vi "Activity_10.vi"() -> ()   [LabVIEW 2015]
panel:
  out "10<Num<30":dbl[](array[numeric])
  out "Array":dbl[](array[numeric])
  out "Num.\nAleatorio":dbl
  out "Iteracion":i32
  # "Selector de números aleatorios en un rango"
  # "Serrano Bermúdez Luis Esteban\nFecha de Entrega 23/02/2019"
  # "Descripción:"
  # "Genera 10 números aleatorios y elige entre un rango de\nvalores determinado (para este ejercicio los valores elegidos\nson 10<Num<30)"
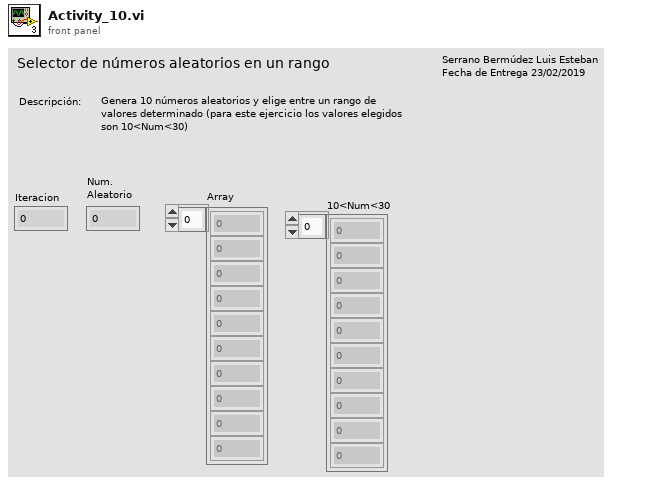
[diagram p1: front panel]
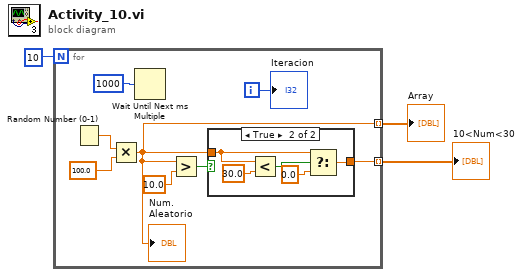
[diagram p0: block diagram]
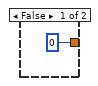
[diagram p2: hidden frame]
diagram:
  n1 = for {
    N: 10 -> [_]
    tunnel: [w5] -> w2 mode=indexing
    tunnel: [w4] -> w1 mode=indexing
    i -> [w11]
    n2 = Random Number (0-1)() -> (number: 0 to 1=w9:dbl)
    n3 = Multiply(x=w9, y=100.0) -> (x*y=w5:dbl)
    "Num.\nAleatorio" <- w5
    n4 = Wait Until Next ms Multiple(millisecond multiple=u32 1000) -> ()  [unwired: 1 out]
    n5 = Greater?(x=w5, y=10.0) -> (0:w6:bool)
    n6 = case shown="True" w6 {
      tunnel: w5 -> [_ w15]
      tunnel: [0 w14] -> w4
      frame False {
      }
      frame True {
        n7 = Less?(x=w15, y=30.0) -> (x < y?=w16:bool)
        n8 = Select(t=w15, s=w16, f=0.0) -> (s? t:f=w14:dbl)
      }
    }
    "Iteracion" <- w11
  }
  "Array" <- w2
  "10<Num<30" <- w1
